vi "Model_Info_and_Report_Data(JSON)(Write).vi"(7 "Dest Folder":path, 8 "error in (no error)":errorcluster, 11 "Model_Info_and_Report":T1={"Name"="", "Feature Extractor"="wrn_50_2_2_bnmerge", "Input3D_Custom_Dims"={"C"=0, "H"=0, "W"=-1}, "Coreset Size"=0, "J-L Proj. Dim."=0, "Train_Time"=0.0, "Inf_Time"=0.0, "Feature_Layers"=[{"Layer_ID"=8, "Patch_Size"=3}, {"Layer_ID"=16, "Patch_Size"=3}], "Eval Stats(Image)"={"Scores(Good)"={"Min"=0.0, "Max"=0.0}, "Scores(Bad)"={"Min"=0.0, "Max"=0.0}, "# of Samples(Good)"=0, "# of Samples(Bad)"=0, "AUROC"=0.0, "F1_Max"=0.0, "Thrshld(F1_Max)"=0.0, "Prec.(F1_Max)"=0.0, "Recall(F1_Max)"=0.0, "FPR(F1_Max)"=0.0, "FNR(F1_Max)"=0.0}, "Eval Stats(Pixel)"={"Scores(Good)"={"Min"=0.0, "Max"=0.0}, "Scores(Bad)"={"Min"=0.0, "Max"=0.0}, "# of Samples(Good)"=0, "# of Samples(Bad)"=0, "AUROC"=0.0, "F1_Max"=0.0, "Thrshld(F1_Max)"=0.0, "Prec.(F1_Max)"=0.0, "Recall(F1_Max)"=0.0, "FPR(F1_Max)"=0.0, "FNR(F1_Max)"=0.0}} {"Eval Stats(Pixel)"."Recall(F1_Max)" format="%#.5f"; "Eval Stats(Pixel)"."FPR(F1_Max)" format="%#.5f"; "Eval Stats(Pixel)"."FNR(F1_Max)" format="%#.5f"; "Eval Stats(Pixel)"."Prec.(F1_Max)" format="%#.5f"; "Eval Stats(Pixel)"."F1_Max" format="%#.5f"; "Eval Stats(Pixel)"."AUROC" format="%#.5f"; "Eval Stats(Pixel)"."Scores(Bad)"."Min" format="%#_5g"; "Eval Stats(Pixel)"."Scores(Good)"."Min" format="%#_5g"; "Eval Stats(Pixel)"."Thrshld(F1_Max)" format="%#_5f"; "Eval Stats(Image)"."Recall(F1_Max)" format="%#.5f"; "Eval Stats(Image)"."FPR(F1_Max)" format="%#.5f"; "Eval Stats(Image)"."FNR(F1_Max)" format="%#.5f"; "Eval Stats(Image)"."Prec.(F1_Max)" format="%#.5f"; "Eval Stats(Image)"."F1_Max" format="%#.5f"; "Eval Stats(Image)"."AUROC" format="%#.5f"; "Eval Stats(Image)"."Scores(Bad)"."Min" format="%#_5g"; "Eval Stats(Image)"."Scores(Good)"."Min" format="%#_5g"; "Eval Stats(Image)"."Thrshld(F1_Max)" format="%#_5f"}) -> (0 "error out":errorcluster, 3 "Generated File Path":path)   [LabVIEW 2020]
uses:
  HyperParam_Investigation/Controls/Model_Info_and_Report.ctl
  <vilib>/Ngene/Deep Learning Toolkit/Toolkit/NN_Data/API/NN_Dims(C,H,W).ctl
  HyperParam_Investigation/Controls/Feature_Layers_CFG.ctl
  <vilib>/Ngene/DeepLTK Anomaly Detection Addon/DeepLTK_Anomaly_Detection_Addon/API/Controls/Eval_Results.ctl
  <vilib>/Ngene/DeepLTK Anomaly Detection Addon/DeepLTK_Anomaly_Detection_Addon/API/Controls/MinMax.ctl
  <vilib>/Ngene/DeepLTK Anomaly Detection Addon/DeepLTK_Anomaly_Detection_Addon/DeepLTK_Anomaly_Detection_Addon.lvlib
  <vilib>/Ngene/Deep Learning Toolkit/Toolkit/Deep_Learning_Toolkit_by_Ngene.lvlib
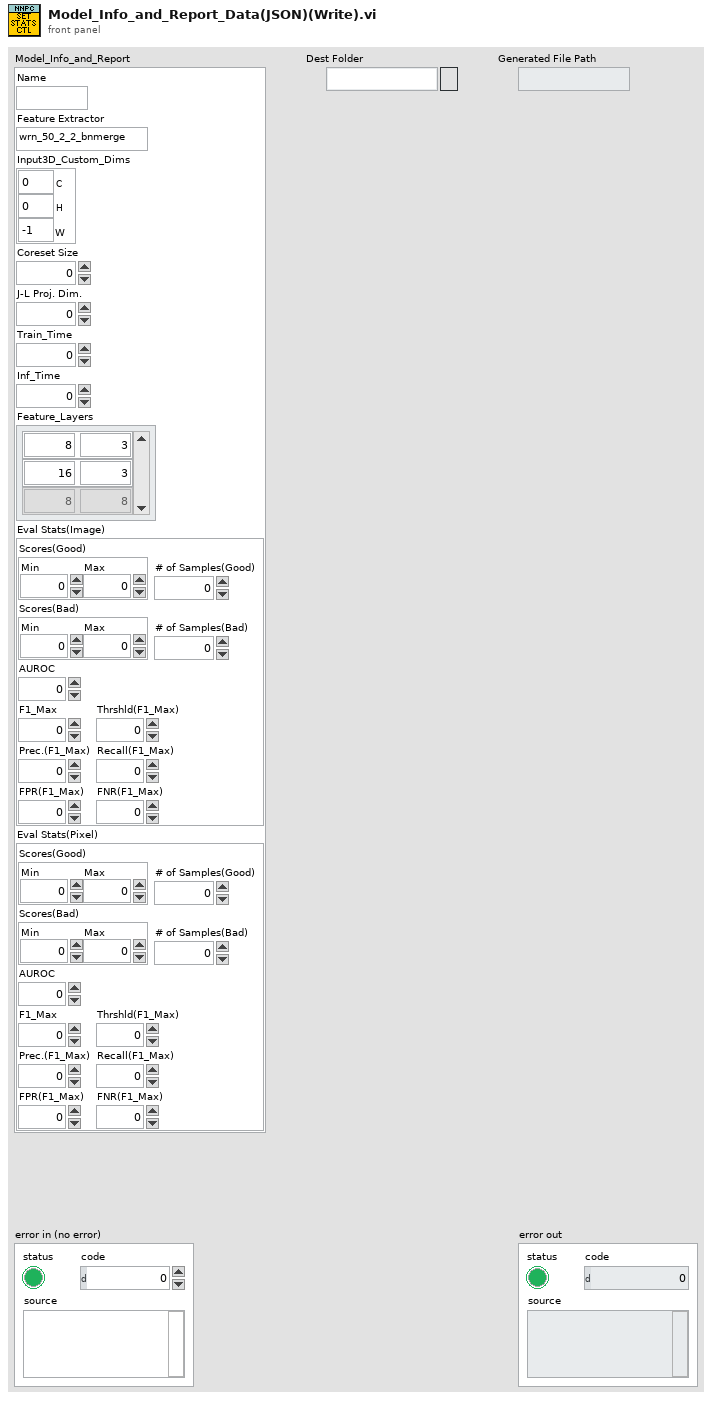
[diagram p1: front panel]
types:
  T1 = typedef "Model_Info_and_Report.ctl" = cluster{"Name":string, "Feature Extractor":string, "Input3D_Custom_Dims":T2, "Coreset Size":i32, "J-L Proj. Dim.":i32, "Train_Time":dbl, "Inf_Time":dbl, "Feature_Layers":T3, "Eval Stats(Image)":T4, "Eval Stats(Pixel)":T4}
  T2 = typedef "Deep_Learning_Toolkit_by_Ngene.lvlib/NN_Dims(C,H,W).ctl" = cluster{"C":i32, "H":i32, "W":i32}
  T3 = typedef "Feature_Layers_CFG.ctl" = cluster{"Layer_ID":i32, "Patch_Size":i32}[]
  T4 = typedef "DeepLTK_Anomaly_Detection_Addon.lvlib/Eval_Results.ctl" = cluster{"Scores(Good)":T5, "Scores(Bad)":T5, "# of Samples(Good)":i32, "# of Samples(Bad)":i32, "AUROC":sgl, "F1_Max":sgl, "Thrshld(F1_Max)":sgl, "Prec.(F1_Max)":sgl, "Recall(F1_Max)":sgl, "FPR(F1_Max)":sgl, "FNR(F1_Max)":sgl}
  T5 = typedef "DeepLTK_Anomaly_Detection_Addon.lvlib/MinMax.ctl" = cluster{"Min":sgl, "Max":sgl}
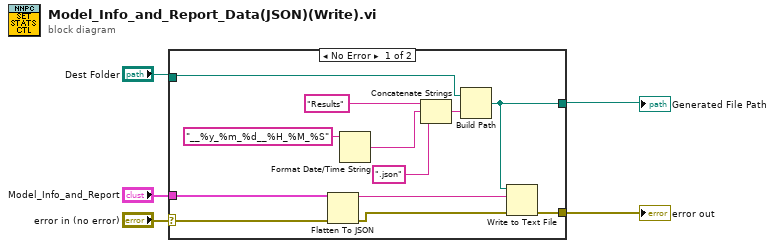
[diagram p0: block diagram]
diagram:
  n1 = case shown="No Error" "error in (no error)" {
    selector: "error in (no error)" -> [w16 w18]
    tunnel: "Model_Info_and_Report" -> [w17 _]
    tunnel: "Dest Folder" -> [w9 _]
    tunnel: [w7 _] -> w2
    tunnel: [w6 w18] -> w1
    frame No Error {
      n2 = Flatten To JSON(anything=w17, error in (no error)=w16) -> (JSON string=w10:string, 11:w8:errorcluster)  [unwired: 1 in]
      n3 = Format Date/Time String(time format string (%c)="__%y_%m_%d__%H_%M_%S") -> (date/time string=w13:string)  [unwired: 2 in]
      n4 = Concatenate Strings("Results" ("string"), w13, ".json" ("string")) -> (w11:string)
      n5 = Build Path(base path=w9, name or relative path=w11) -> (appended path=w7:path)
      n6 = Write to Text File(file (use dialog)=w7, text=w10, error in=w8) -> (error out=w6:errorcluster)  [unwired: 1 in, 2 out]
    }
    frame Error {
    }
  }
  "Generated File Path" <- w2
  "error out" <- w1
